vi "Main.vi"() -> ()   [LabVIEW 2018]
panel:
  out "Write Read Time":u32
  out "Total Time":u32
  out "data out":string
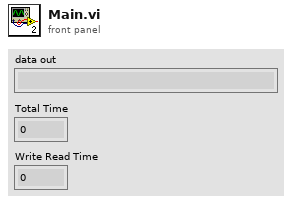
[diagram p1: front panel]
types:
  T1 = enum16{"Standard", "Buffered", "CRLF", "Immediate"}
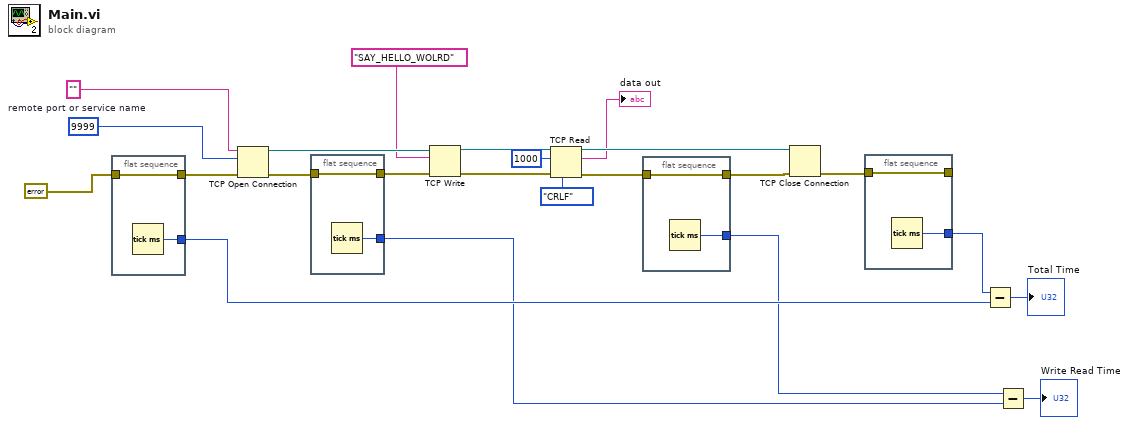
[diagram p0: block diagram]
diagram:
  w12 = u16 9999  # remote port or service name
  n1 = flat-sequence {
    tunnel: errorcluster {"status"=FALSE, "code"=0, "source"=""} ("error in (no error)") -> [w25]
    tunnel: [w25] -> w13
    tunnel: [w24] -> w11
    frame #0 {
      n2 = Tick Count (ms)() -> (millisecond timer value=w24:u32)
    }
  }
  n3 = TCP Open Connection(address="", remote port or service name=w12, error in (no error)=w13) -> (connection ID=w23:refnum<k5>, error out=w9:errorcluster)  [unwired: 2 in]
  n4 = flat-sequence {
    tunnel: w9 -> [w27]
    tunnel: [w27] -> w8
    tunnel: [w26] -> w1
    frame #0 {
      n5 = Tick Count (ms)() -> (millisecond timer value=w26:u32)
    }
  }
  n6 = TCP Write(connection ID=w23, data in="SAY_HELLO_WOLRD", error in (no error)=w8) -> (connection ID out=w22:refnum<k5>, error out=w15:errorcluster)  [unwired: 1 in, 1 out]
  n7 = TCP Read(connection ID=w22, bytes to read=1000, error in (no error)=w15, 7:T1."CRLF" ("mode (standard)")) -> (connection ID out=w21:refnum<k5>, data out=→"data out":string, error out=w4:errorcluster)  [unwired: 1 in]
  n8 = flat-sequence {
    tunnel: w4 -> [w29]
    tunnel: [w29] -> w3
    tunnel: [w28] -> w2
    frame #0 {
      n9 = Tick Count (ms)() -> (millisecond timer value=w28:u32)
    }
  }
  n10 = TCP Close Connection(connection ID=w21, error in (no error)=w3) -> (error out=w7:errorcluster)  [unwired: 1 in, 1 out]
  n11 = flat-sequence {
    tunnel: w7 -> [w31]
    tunnel: [w31] -> _
    tunnel: [w30] -> w6
    frame #0 {
      n12 = Tick Count (ms)() -> (millisecond timer value=w30:u32)
    }
  }
  n13 = Subtract(x=w6, y=w11) -> (x-y=→"Total Time":u32)
  n14 = Subtract(x=w2, y=w1) -> (x-y=→"Write Read Time":u32)
